vi "Process Messages.vi"(8 "error in (no error)":errorcluster, 11 "Deck in":refnum<class "Deck.lvclass">) -> (0 "error out":errorcluster, 3 "Deck out":refnum<class "Deck.lvclass">)   [LabVIEW 2018, in "Deck.lvclass"]
uses:
  Deck.lvclass
  Deck.lvclass/Deck.ctl
  State.ctl
  Libraries/Messaging/Message Cluster.ctl
  Libraries/Track Info/Track Info.ctl
  Libraries/Audio Processing/Value Properties.ctl
  Libraries/Track Info/Track Info FGV Enum.ctl
  d748f491-0a50-4902-99a1-0e4baec2160f.vi
  Libraries/Globals/Constants.vi
  Libraries/Audio Input/Audio File Input.lvlib
  Libraries/Messaging/Messaging.lvlib
  Libraries/User Interface/User Interface.lvlib
  Libraries/Track Info/Track Info.lvlib
  Libraries/Globals/Globals.lvlib
  Libraries/Audio Processing/Audio Processing.lvlib
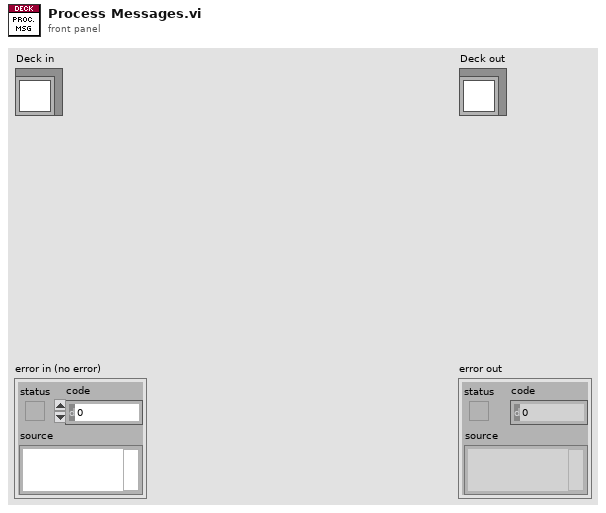
[diagram p1: front panel]
types:
  T1 = typedef "Messaging.lvlib/Message Cluster.ctl" = cluster{"Event":string, "Source":string, "Target":string, "Data":variant}
  T2 = typedef "Deck.lvclass/State.ctl" = enum16{"No Track", "Loading", "Active", "Scratching", "Brake", "Backspin"}
  T3 = typedef "Track Info.lvlib/Track Info.ctl" = cluster{"Path":path, "Length (Samples)":i32, "Channels":i32, "Sample Rate (Hz)":i32, "BPM":dbl, "Cue Points (Samples)":i32[]}
  T4 = typedef "Audio Processing.lvlib/Value Properties.ctl" = cluster{"Lower":dbl, "Upper":dbl}
  T5 = typedef "Track Info.lvlib/Track Info FGV Enum.ctl" = enum16{"Init", "Update Track", "Update Multiple Tracks", "Get Track", "Get Multiple Tracks"}
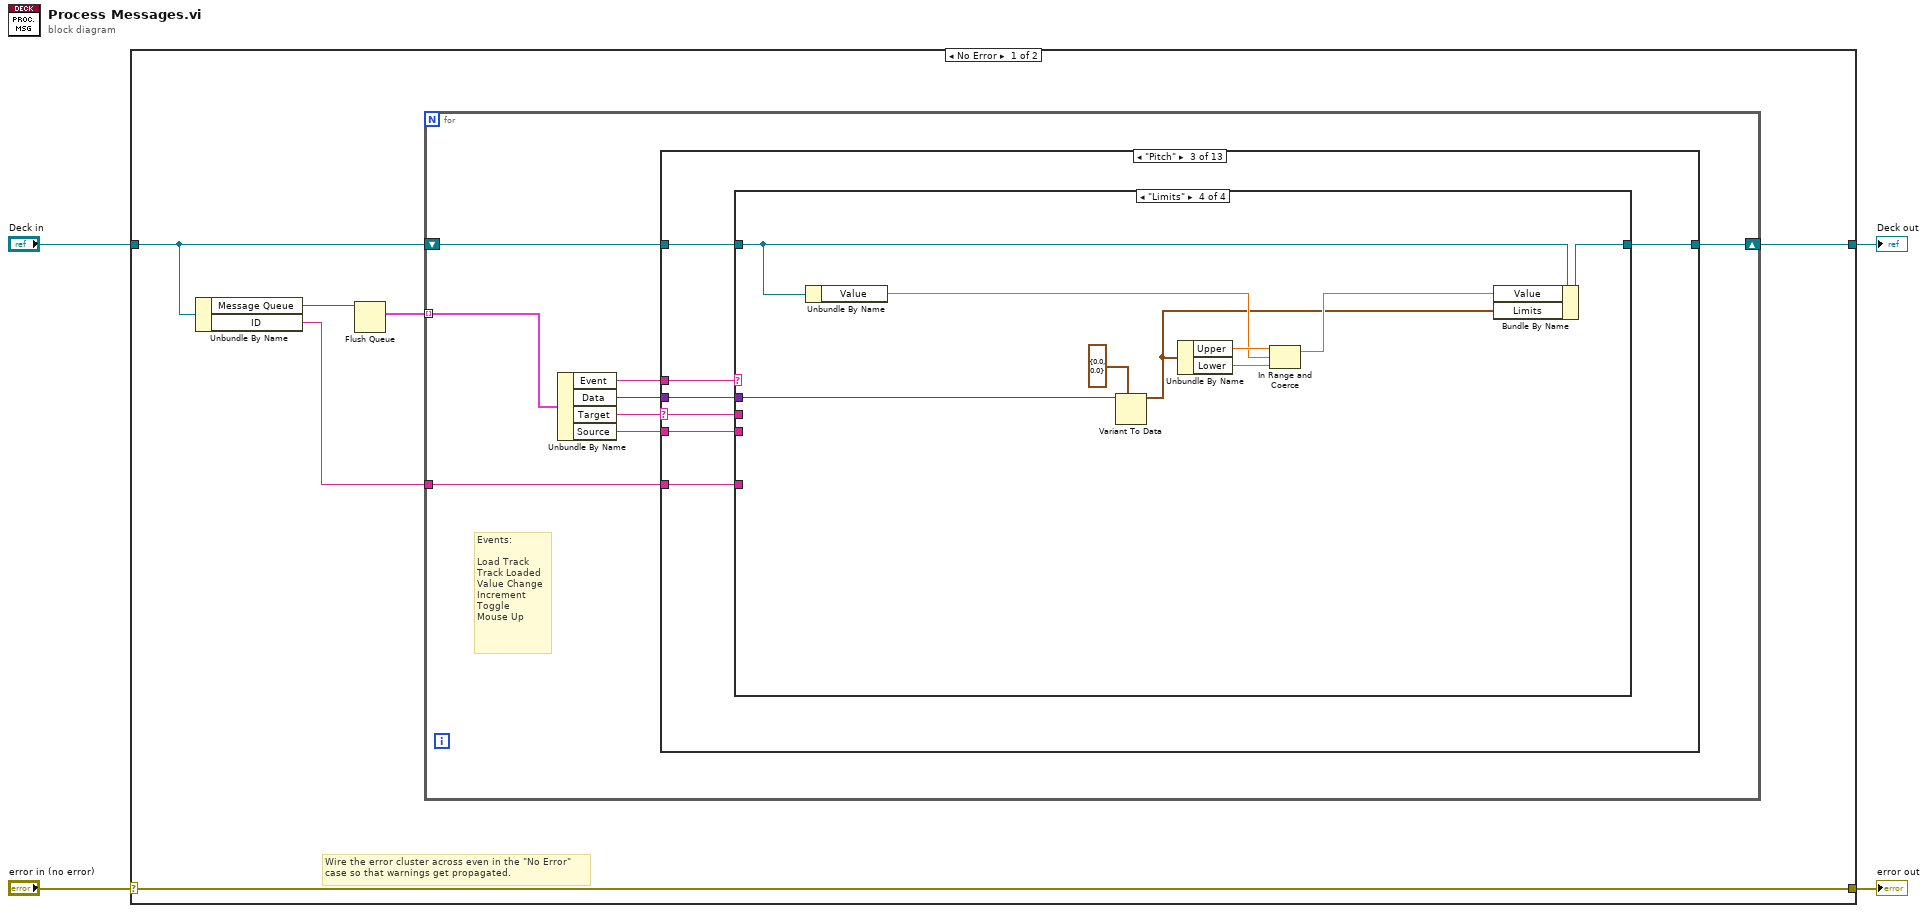
[diagram p0: block diagram]
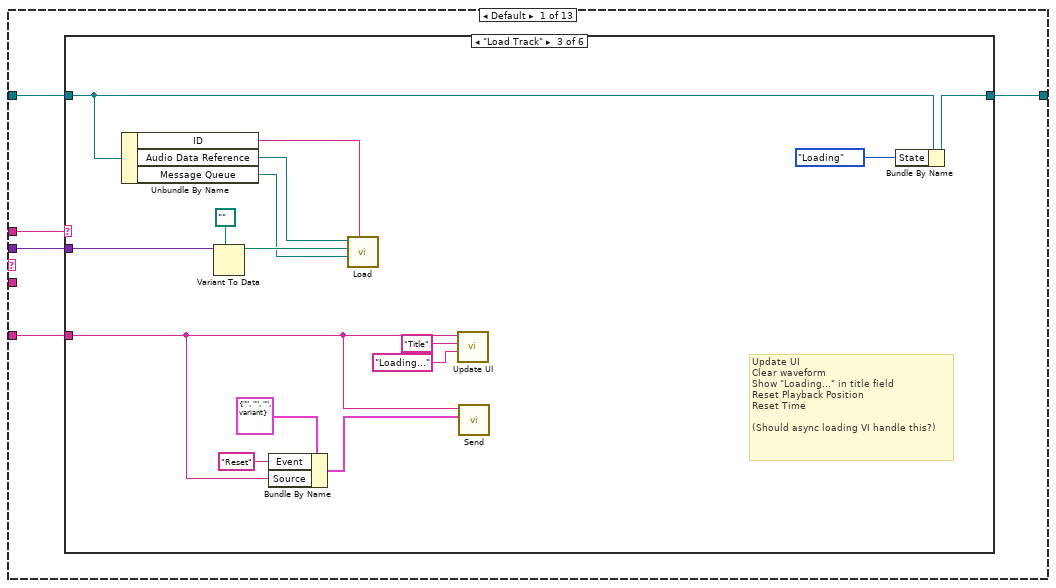
[diagram p2: hidden frame]
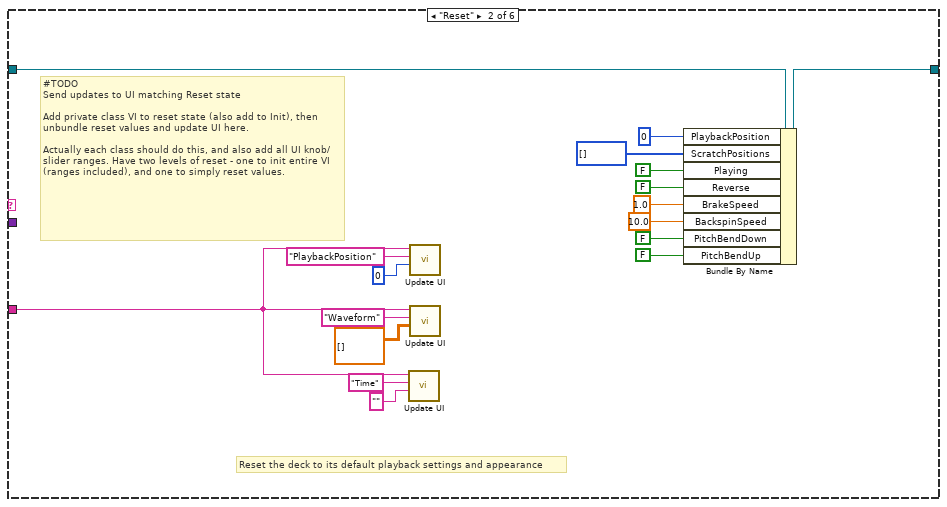
[diagram p4: hidden frame]
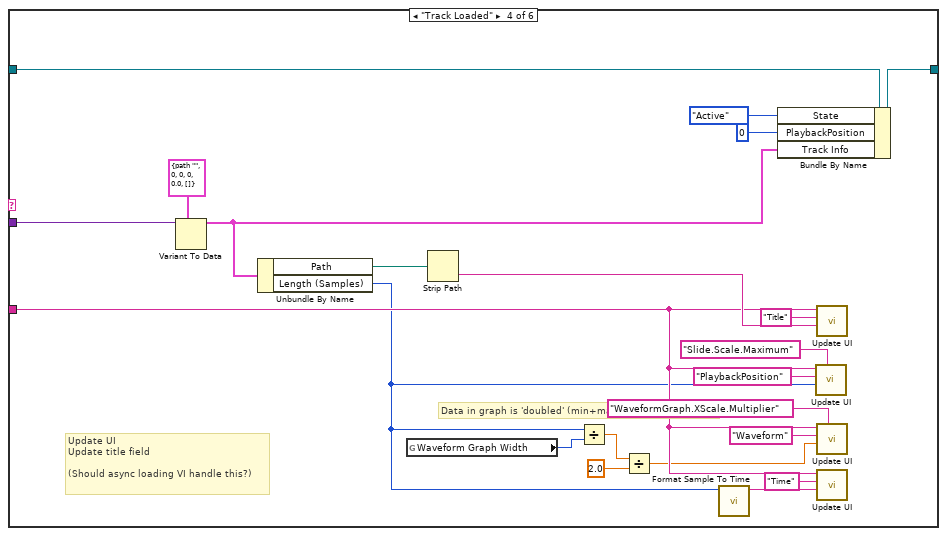
[diagram p5: hidden frame]
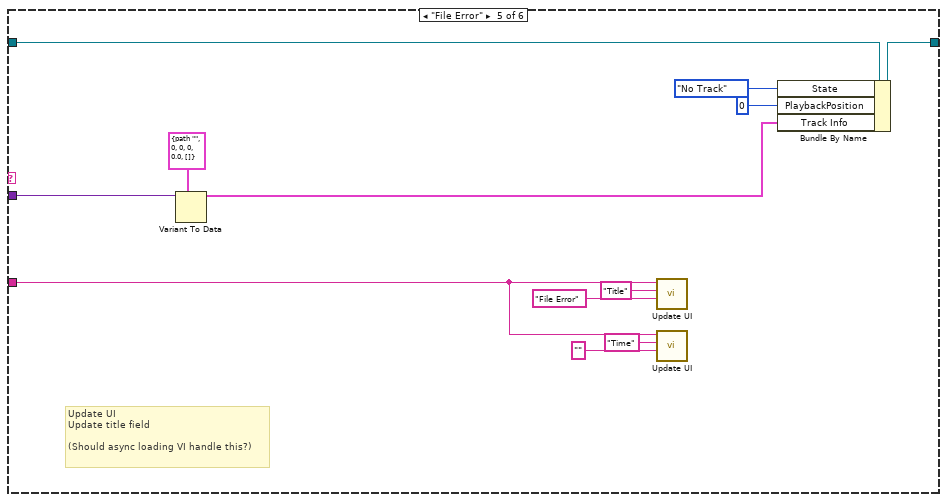
[diagram p6: hidden frame]
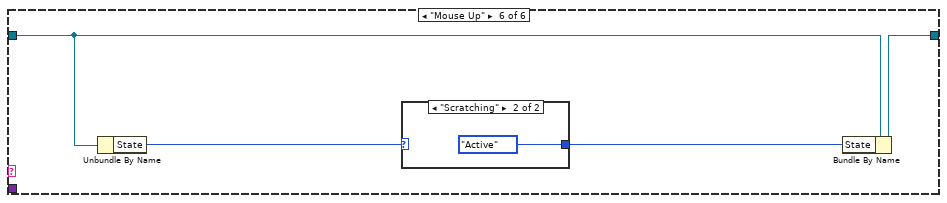
[diagram p7: hidden frame]
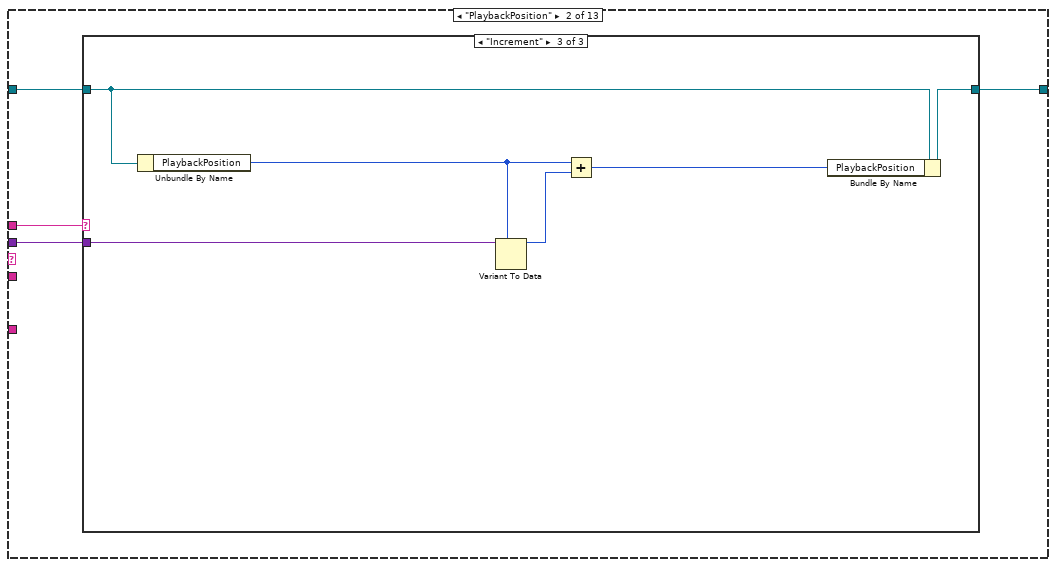
[diagram p9: hidden frame]
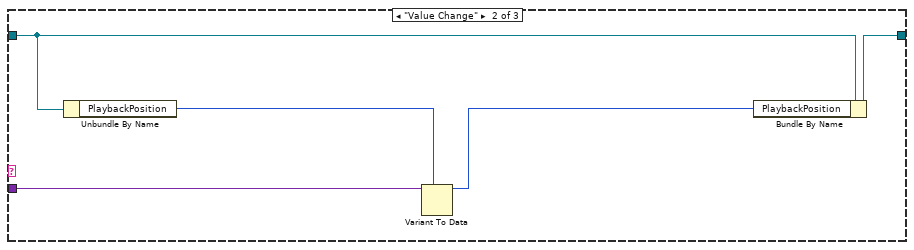
[diagram p11: hidden frame]
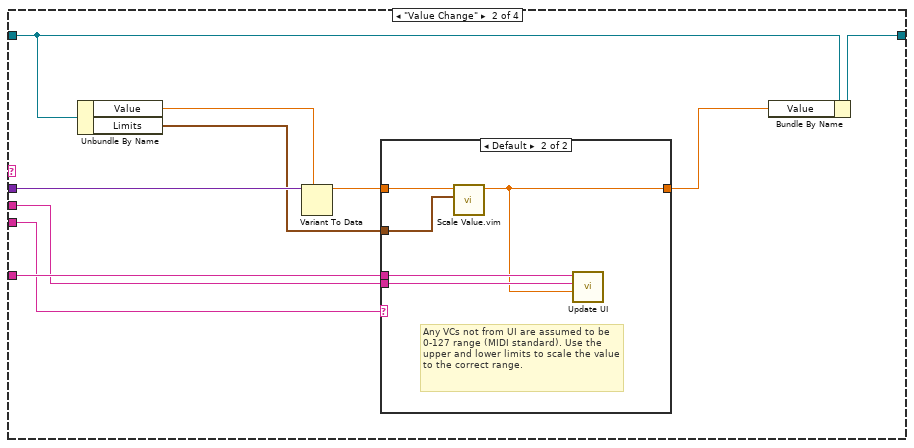
[diagram p13: hidden frame]
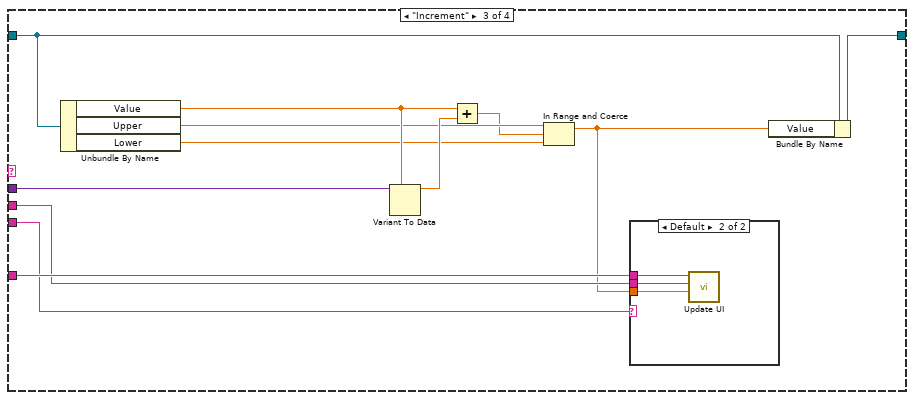
[diagram p15: hidden frame]
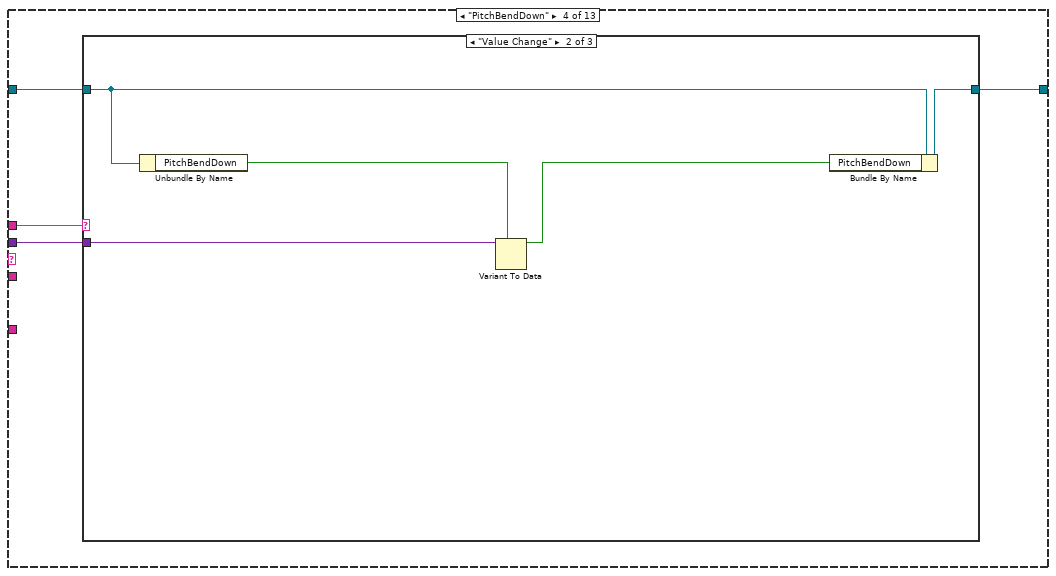
[diagram p17: hidden frame]
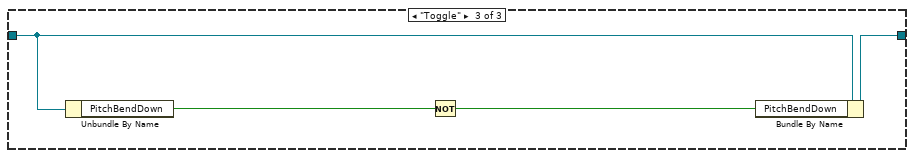
[diagram p19: hidden frame]
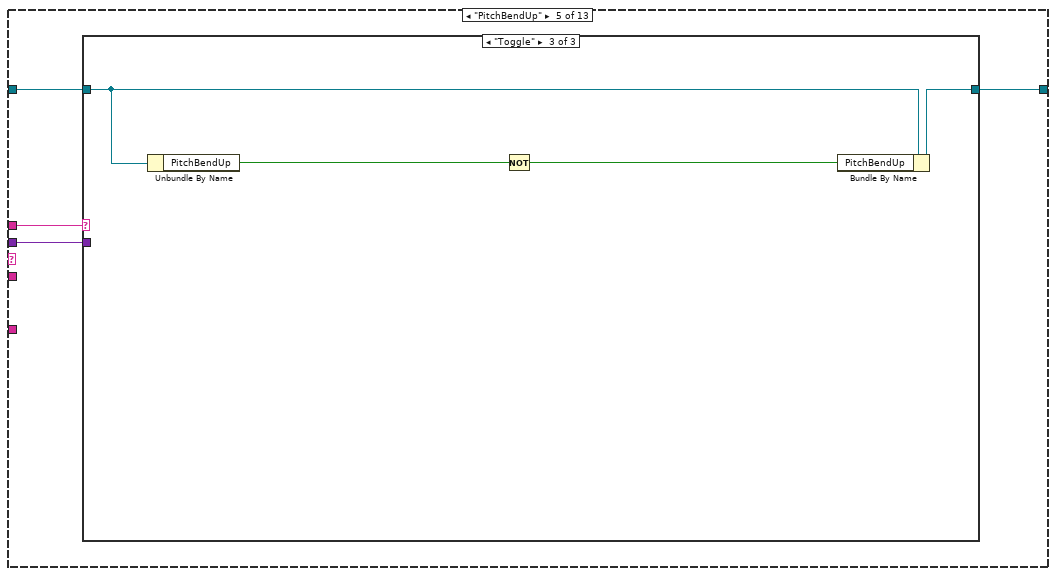
[diagram p20: hidden frame]
diagram:
  n1 = case shown="No Error" "error in (no error)" {
    selector: "error in (no error)" -> [w10 w528]
    tunnel: [w10 w528] -> w3
    tunnel: [w9 w527] -> w1
    tunnel: "Deck in" -> [w8 w527]
    frame No Error {
      # "Wire the error cluster across even in the \"No Error\"\ncase so that warnings get propagated."
      n2 = Unbundle By Name(w8) -> ("Message Queue"=w6:refnum<queue>, "ID"=w7:string)
      n3 = Flush Queue(queue=w6) -> (remaining elements=w5:T1[])  [unwired: 1 in, 2 out]
      n4 = for {
        shift-right: [w16] -> w9
        shift-left: w8 -> [w18]
        tunnel: w7 -> [w14]
        tunnel: w5 -> [w11] mode=indexing
        # "Events:\n\nLoad Track\nTrack Loaded\nValue Change\nIncrement\nToggle\nMouse Up"
        n5 = Unbundle By Name(w11) -> ("Event"=w17:string, "Data"=w15:variant, "Target"=w13:string, "Source"=w12:string)
        n6 = case shown="\"Pitch\"" w13 {
          selector: w13 -> [_ _ w114 _ _ _ w208 w239 w260 w280 w317 w347 w438]
          tunnel: w18 -> [w23 w100 w119 w164 w178 w192 w213 w243 w264 w284 w322 w351 w442]
          tunnel: w17 -> [w22 w99 w118 w163 w177 w191 w212 w242 w263 w283 w321 w350 w441]
          tunnel: [w21 w98 w117 w162 w176 w190 w211 w241 w262 w282 w320 w349 w440] -> w16
          tunnel: w15 -> [w20 w97 w116 w161 w175 w189 w210 w240 w261 w281 w319 w348 w439]
          tunnel: w14 -> [w19 _ w115 _ _ _ w209 w238 _ w279 w318 w346 w437]
          tunnel: w12 -> [_ _ w113 _ _ _ _ _ _ w278 w316 w345 w436]
          frame Default {
            n7 = case shown="\"Load Track\"" w22 {
              tunnel: w23 -> [w24 w33 w49 w76 w88 w91]
              tunnel: [w24 w34 w50 w75 w87 w92] -> w21
              tunnel: w20 -> [_ _ w48 w74 w86 _]
              tunnel: w19 -> [_ w35 w43 w62 w82 _]
              frame Default {
              }
              frame "Reset" {
                # "#TODO\nSend updates to UI matching Reset state\n\nAdd private class VI to reset state (also add to Init), then unbundle reset values and update UI here.\n\nActually each class should do this, and also add all UI knob/slider ranges. Have two levels of reset - one to init entire VI (ranges included), and one to simply reset values."
                # "Reset the deck to its default playback settings and appearance"
                n8 = call "Update UI.vi"("Data"="" ("Target"), "Target"="Time", "ID"=w35) -> ()  [unwired: 8 in, 1 out]
                n9 = call "Update UI.vi"("Data"=0, "Target"="PlaybackPosition", "ID"=w35) -> ()  [unwired: 8 in, 1 out]
                n10 = call "Update UI.vi"("Data"=dbl[][] [], "Target"="Waveform", "ID"=w35) -> ()  [unwired: 8 in, 1 out]
                n11 = Bundle By Name(cluster=w33, "PlaybackPosition"=0, "ScratchPositions"=i32[] [], "Playing"=FALSE, "Reverse"=FALSE, "BrakeSpeed"=1.0, "BackspinSpeed"=10.0, "PitchBendDown"=FALSE, "PitchBendUp"=FALSE) -> (w34:refnum<class "Deck.lvclass">)
              }
              frame "Load Track" {
                # "Update UI\nClear waveform\nShow \"Loading...\" in title field\nReset Playback Position\nReset Time\n\n(Should async loading VI handle this?)"
                n12 = Unbundle By Name(w49) -> ("ID"=w56:string, "Audio Data Reference"=w53:refnum<data-value>, "Message Queue"=w52:refnum<queue>)
                n13 = Variant To Data(type=path "", Variant=w48) -> (data=w55:path)  [unwired: 1 in, 1 out]
                n14 = Bundle By Name(cluster=T1 {"Event"="", "Source"="", "Target"="", "Data"=variant} ("Message"), "Event"="Reset", "Source"=w43) -> (w42:T1)
                n15 = call "Load.vi"("Deck ID"=w56, "Message Queue"=w52, "Path"=w55, "Audio Data Reference"=w53) -> ()  [unwired: 7 in, 1 out]
                n16 = call "Update UI.vi"("Data"="Loading..." ("Target"), "Target"="Title", "ID"=w43) -> ()  [unwired: 8 in, 1 out]
                n17 = call "Send.vi"("Message"=w42, "Queue Name"=w43) -> ()  [unwired: 9 in, 1 out]
                n18 = Bundle By Name(cluster=w49, "State"=State."Loading") -> (w50:refnum<class "Deck.lvclass">)
              }
              frame "Track Loaded" {
                # "Data in graph is 'doubled' (min+max for every point)"
                # "Update UI\nUpdate title field\n\n(Should async loading VI handle this?)"
                n19 = Variant To Data(type=T3 {"Path"=path "", "Length (Samples)"=0, "Channels"=0, "Sample Rate (Hz)"=0, "BPM"=0.0, "Cue Points (Samples)"=[]} ("Track Info"), Variant=w74) -> (data=w72:T3)  [unwired: 1 in, 1 out]
                n20 = Unbundle By Name(w72) -> ("Path"=w71:path, "Length (Samples)"=w61:i32)
                n21 = global read "Constants.vi" "Waveform Graph Width"() -> (w60:i32)
                n22 = Strip Path(path=w71) -> (name=w70:string)  [unwired: 1 out]
                n23 = Divide(x=w61, y=w60) -> (x/y=w59:dbl)
                n24 = Divide(x=w59, y=2.0 ("x")) -> (x/y=w57:dbl)
                n25 = call "Format Sample To Time.vi"("Samples"=w61) -> ("Formatted Time"=w66:string)  [unwired: 10 in]
                n26 = Bundle By Name(cluster=w76, "State"=State."Active", "PlaybackPosition"=0 ("Playback Position (Samples)"), "Track Info"=w72) -> (w75:refnum<class "Deck.lvclass">)
                n27 = call "Update UI.vi"("Message (Value Change)"="Slide.Scale.Maximum" ("Target"), "Data"=w61, "Target"="PlaybackPosition", "ID"=w62) -> ()  [unwired: 7 in, 1 out]
                n28 = call "Update UI.vi"("Data"=w70, "Target"="Title", "ID"=w62) -> ()  [unwired: 8 in, 1 out]
                n29 = call "Update UI.vi"("Message (Value Change)"="WaveformGraph.XScale.Multiplier" ("Target"), "Data"=w57, "Target"="Waveform", "ID"=w62) -> ()  [unwired: 7 in, 1 out]
                n30 = call "Update UI.vi"("Data"=w66, "Target"="Time", "ID"=w62) -> ()  [unwired: 8 in, 1 out]
              }
              frame "File Error" {
                # "Update UI\nUpdate title field\n\n(Should async loading VI handle this?)"
                n31 = Variant To Data(type=T3 {"Path"=path "", "Length (Samples)"=0, "Channels"=0, "Sample Rate (Hz)"=0, "BPM"=0.0, "Cue Points (Samples)"=[]} ("Track Info"), Variant=w86) -> (data=w84:T3)  [unwired: 1 in, 1 out]
                n32 = call "Update UI.vi"("Data"="File Error" ("Target"), "Target"="Title", "ID"=w82) -> ()  [unwired: 8 in, 1 out]
                n33 = call "Update UI.vi"("Data"="" ("Target"), "Target"="Time", "ID"=w82) -> ()  [unwired: 8 in, 1 out]
                n34 = Bundle By Name(cluster=w88, "State"=State."No Track", "PlaybackPosition"=0 ("Playback Position (Samples)"), "Track Info"=w84) -> (w87:refnum<class "Deck.lvclass">)
              }
              frame "Mouse Up" {
                n35 = Unbundle By Name(w91) -> ("State"=w93:T2)
                n36 = case shown="\"Scratching\"" w93 {
                  selector: w93 -> [w95 _]
                  tunnel: [w95 State."Active" ("State")] -> w94
                  frame Default {
                  }
                  frame "Scratching" {
                  }
                }
                n37 = Bundle By Name(cluster=w91, "State"=w94) -> (w92:refnum<class "Deck.lvclass">)
              }
            }
          }
          frame "PlaybackPosition" {
            n38 = case shown="\"Increment\"" w99 {
              tunnel: w100 -> [w101 w105 w111]
              tunnel: [w101 w106 w112] -> w98
              tunnel: w97 -> [_ w103 w110]
              frame Default {
              }
              frame "Value Change" {
                n39 = Unbundle By Name(w105) -> ("PlaybackPosition"=w104:i32)
                n40 = Variant To Data(type=w104, Variant=w103) -> (data=w102:i32)  [unwired: 1 in, 1 out]
                n41 = Bundle By Name(cluster=w105, "PlaybackPosition"=w102) -> (w106:refnum<class "Deck.lvclass">)
              }
              frame "Increment" {
                n42 = Unbundle By Name(w111) -> ("PlaybackPosition"=w109:i32)
                n43 = Variant To Data(type=w109, Variant=w110) -> (data=w108:i32)  [unwired: 1 in, 1 out]
                n44 = Add(x=w109, y=w108) -> (x+y=w107:i32)
                n45 = Bundle By Name(cluster=w111, "PlaybackPosition"=w107) -> (w112:refnum<class "Deck.lvclass">)
              }
            }
          }
          frame "Pitch" {
            n46 = case shown="\"Limits\"" w118 {
              tunnel: w119 -> [w120 w129 w147 w159]
              tunnel: [w120 w130 w148 w160] -> w117
              tunnel: w116 -> [_ w127 w146 w158]
              tunnel: w115 -> [_ w126 w143 _]
              tunnel: w114 -> [_ w124 w142 _]
              tunnel: w113 -> [_ w123 w141 _]
              frame Default {
              }
              frame "Value Change" {
                n47 = Unbundle By Name(w129) -> ("Value"=w128:dbl, "Limits"=w121:T4)
                n48 = Variant To Data(type=w128, Variant=w127) -> (data=w125:dbl)  [unwired: 1 in, 1 out]
                n49 = case shown="Default" w123 {
                  tunnel: w126 -> [_ w136]
                  tunnel: w124 -> [_ w135]
                  tunnel: w125 -> [w131 w132]
                  tunnel: [w131 w133] -> w122
                  tunnel: w121 -> [_ w134]
                  frame "UI" {
                    # "VC from UI are assumed to be in range."
                  }
                  frame Default {
                    # "Any VCs not from UI are assumed to be 0-127 range (MIDI standard). Use the upper and lower limits to scale the value to the correct range."
                    n50 = call "Scale Value.vim"("Limits"=w134, "Value"=w132) -> ("Scaled Value"=w133:dbl)  [unwired: 9 in]
                    n51 = call "Update UI.vi"("Data"=w133, "Target"=w135, "ID"=w136) -> ()  [unwired: 8 in, 1 out]
                  }
                }
                n52 = Bundle By Name(cluster=w129, "Value"=w122) -> (w130:refnum<class "Deck.lvclass">)
              }
              frame "Increment" {
                n53 = Unbundle By Name(w147) -> ("Value"=w145:dbl, "Upper"=w140:dbl, "Lower"=w139:dbl)
                n54 = Variant To Data(type=w145, Variant=w146) -> (data=w144:dbl)  [unwired: 1 in, 1 out]
                n55 = Add(x=w145, y=w144) -> (x+y=w138:dbl)
                n56 = In Range and Coerce(upper limit=w140, x=w138, lower limit=w139) -> (coerced(x)=w137:dbl)  [unwired: 1 out]
                n57 = case shown="Default" w141 {
                  tunnel: w143 -> [_ w151]
                  tunnel: w142 -> [_ w150]
                  tunnel: w137 -> [_ w149]
                  frame "UI" {
                  }
                  frame Default {
                    n58 = call "Update UI.vi"("Data"=w149, "Target"=w150, "ID"=w151) -> ()  [unwired: 8 in, 1 out]
                  }
                }
                n59 = Bundle By Name(cluster=w147, "Value"=w137) -> (w148:refnum<class "Deck.lvclass">)
              }
              frame "Limits" {
                n60 = Unbundle By Name(w159) -> ("Value"=w153:dbl)
                n61 = Variant To Data(type=T4 {"Lower"=0.0, "Upper"=0.0} ("Value Properties"), Variant=w158) -> (data=w152:T4)  [unwired: 1 in, 1 out]
                n62 = Unbundle By Name(w152) -> ("Upper"=w155:dbl, "Lower"=w154:dbl)
                n63 = In Range and Coerce(upper limit=w155, x=w153, lower limit=w154) -> (coerced(x)=w157:dbl)  [unwired: 1 out]
                n64 = Bundle By Name(cluster=w159, "Value"=w157, "Limits"=w152) -> (w160:refnum<class "Deck.lvclass">)
              }
            }
          }
          frame "PitchBendDown" {
            n65 = case shown="\"Value Change\"" w163 {
              tunnel: w164 -> [w165 w169 w173]
              tunnel: [w165 w170 w174] -> w162
              tunnel: w161 -> [_ w167 _]
              frame Default {
              }
              frame "Value Change" {
                n66 = Unbundle By Name(w169) -> ("PitchBendDown"=w168:bool)
                n67 = Variant To Data(type=w168, Variant=w167) -> (data=w166:bool)  [unwired: 1 in, 1 out]
                n68 = Bundle By Name(cluster=w169, "PitchBendDown"=w166) -> (w170:refnum<class "Deck.lvclass">)
              }
              frame "Toggle" {
                n69 = Unbundle By Name(w173) -> ("PitchBendDown"=w172:bool)
                n70 = Not(x=w172) -> (.not. x?=w171:bool)
                n71 = Bundle By Name(cluster=w173, "PitchBendDown"=w171) -> (w174:refnum<class "Deck.lvclass">)
              }
            }
          }
          frame "PitchBendUp" {
            n72 = case shown="\"Toggle\"" w177 {
              tunnel: w178 -> [w179 w183 w187]
              tunnel: [w179 w184 w188] -> w176
              tunnel: w175 -> [_ w181 _]
              frame Default {
              }
              frame "Value Change" {
                n73 = Unbundle By Name(w183) -> ("PitchBendUp"=w182:bool)
                n74 = Variant To Data(type=w182, Variant=w181) -> (data=w180:bool)  [unwired: 1 in, 1 out]
                n75 = Bundle By Name(cluster=w183, "PitchBendUp"=w180) -> (w184:refnum<class "Deck.lvclass">)
              }
              frame "Toggle" {
                n76 = Unbundle By Name(w187) -> ("PitchBendUp"=w186:bool)
                n77 = Not(x=w186) -> (.not. x?=w185:bool)
                n78 = Bundle By Name(cluster=w187, "PitchBendUp"=w185) -> (w188:refnum<class "Deck.lvclass">)
              }
            }
          }
          frame "Jogwheel" {
            n79 = case shown="\"Value Change\"" w191 {
              tunnel: w192 -> [w193 w204]
              tunnel: [w193 w205] -> w190
              tunnel: w189 -> [_ w203]
              frame Default {
              }
              frame "Value Change" {
                n80 = Unbundle By Name(w204) -> ("State"=w202:T2, "ScratchPositions"=w199:i32[], "PlaybackPosition"=w197:i32)
                n81 = Variant To Data(type=w197, Variant=w203) -> (data=w196:i32)  [unwired: 1 in, 1 out]
                n82 = Subtract(x=w199, y=w197) -> (x-y=w200:i32[])
                n83 = case shown="\"Active\"" w202 {
                  selector: w202 -> [w206 _]
                  tunnel: [w206 State."Scratching" ("State")] -> w201
                  frame Default {
                  }
                  frame "Active" {
                  }
                }
                n84 = Add Array Elements(numeric array=w200) -> (sum=w198:i32)
                n85 = Compound Arithmetic op=ADD(w198, w197, w196) -> (w195:i32)
                n86 = Build Array(w195) -> (w194:i32[])
                n87 = Bundle By Name(cluster=w204, "State"=w201, "ScratchPositions"=w194) -> (w205:refnum<class "Deck.lvclass">)
              }
            }
          }
          frame "Cue1", "Cue2", "Cue3" {
            n88 = case shown="\"Value Change\"" w212 {
              tunnel: w213 -> [w214 w225]
              tunnel: [w214 w226] -> w211
              tunnel: w210 -> [_ _]
              tunnel: w209 -> [_ w221]
              tunnel: w208 -> [_ w217]
              frame Default {
              }
              frame "Value Change" {
                n89 = Unbundle By Name(w225) -> ("Cue Points (Samples)"=w224:i32[], "Length (Samples)"=w220:i32)
                n90 = Reverse String(1:w217) -> (0:w219:string)
                n91 = Scan From String(format string="%d", input string=w219) -> (output 1=w216:i32)  [unwired: 3 in, 3 out]
                n92 = Decrement(x=w216) -> (x-1=w215:i32)
                n93 = Index Array(array=w224, index=w215) -> (element=w222:i32)
                n94 = Greater Or Equal To 0?(x=w222) -> (x >= 0?=w223:bool)
                n95 = case shown="True" w223 {
                  tunnel: [w227 w237] -> w226
                  tunnel: w225 -> [w227 w236]
                  tunnel: w222 -> [_ w229]
                  tunnel: w221 -> [_ w230]
                  tunnel: w220 -> [_ w231]
                  frame False {
                  }
                  frame True {
                    n96 = Subtract(x=w231, y=w229) -> (x-y=w228:i32)
                    n97 = call "Format Sample To Time.vi"("Samples"=w228) -> ("Formatted Time"=w235:string)  [unwired: 10 in]
                    n98 = Bundle By Name(cluster=w236, "PlaybackPosition"=w229) -> (w237:refnum<class "Deck.lvclass">)
                    n99 = call "Update UI.vi"("Data"=w229, "Target"="PlaybackPosition" ("format string"), "ID"=w230) -> ()  [unwired: 8 in, 1 out]
                    n100 = call "Update UI.vi"("Data"=w229, "Target"="Jogwheel" ("format string"), "ID"=w230) -> ()  [unwired: 8 in, 1 out]
                    n101 = call "Update UI.vi"("Data"=w235, "Target"="Time" ("format string"), "ID"=w230) -> ()  [unwired: 8 in, 1 out]
                  }
                }
              }
            }
          }
          frame "SetCue1", "SetCue2", "SetCue3" {
            n102 = case shown="\"Value Change\"" w242 {
              tunnel: w243 -> [w244 w259]
              tunnel: [w244 w255] -> w241
              tunnel: w240 -> [_ _]
              tunnel: w239 -> [_ w253]
              tunnel: w238 -> [_ w246]
              frame Default {
              }
              frame "Value Change" {
                n103 = Unbundle By Name(w259) -> ("PlaybackPosition"=w258:i32, "Cue Points (Samples)"=w254:i32[])
                n104 = Reverse String(1:w253) -> (0:w252:string)
                n105 = Scan From String(format string="%d", input string=w252) -> (output 1=w250:i32)  [unwired: 3 in, 3 out]
                n106 = Decrement(x=w250) -> (x-1=w249:i32)
                n107 = Replace Array Subset(array=w254, new element=w258, index=w249) -> (w247:i32[])
                n108 = Bundle By Name(cluster=w259, "Cue Points (Samples)"=w247) -> (w255:refnum<class "Deck.lvclass">)
                n109 = call "Update UI.vi"("Message (Value Change)"="WaveformGraph.Cues" ("format string"), "Data"=w247, "Target"="Waveform", "ID"=w246) -> ()  [unwired: 7 in, 1 out]
                n110 = Unbundle By Name(w255) -> ("Track Info"=w257:T3)
                n111 = call "Track Info FGV.vi"("Track Info FGV Enum"=Track_Info_FGV_Enum."Update Track", "Track Info In"=w257) -> ()  [unwired: 6 in, 4 out]
              }
            }
          }
          frame "ClearCue1", "ClearCue2", "ClearCue3" {
            n112 = case shown="\"Value Change\"" w263 {
              tunnel: w264 -> [w265 w277]
              tunnel: [w265 w266] -> w262
              tunnel: w261 -> [_ _]
              tunnel: w260 -> [_ w269]
              frame Default {
              }
              frame "Value Change" {
                n113 = Unbundle By Name(w277) -> ("Cue Points (Samples)"=w276:i32[])
                n114 = Reverse String(1:w269) -> (0:w271:string)
                n115 = Scan From String(format string="%d", input string=w271) -> (output 1=w268:i32)  [unwired: 3 in, 3 out]
                n116 = Decrement(x=w268) -> (x-1=w267:i32)
                n117 = Replace Array Subset(array=w276, new element=-2147483648 ("new element/subarray"), index=w267) -> (w275:i32[])
                n118 = Bundle By Name(cluster=w277, "Cue Points (Samples)"=w275) -> (w266:refnum<class "Deck.lvclass">)
                n119 = Unbundle By Name(w266) -> ("Track Info"=w273:T3)
                n120 = call "Track Info FGV.vi"("Track Info FGV Enum"=Track_Info_FGV_Enum."Update Track", "Track Info In"=w273) -> ()  [unwired: 6 in, 4 out]
              }
            }
          }
          frame "Play" {
            n121 = case shown="\"Value Change\"" w283 {
              tunnel: w284 -> [w285 w293 w308]
              tunnel: [w285 w294 w309] -> w282
              tunnel: w281 -> [_ w291 _]
              tunnel: w280 -> [_ w289 w305]
              tunnel: w279 -> [_ w288 w304]
              tunnel: w278 -> [_ w287 w302]
              frame Default {
              }
              frame "Value Change" {
                n122 = Unbundle By Name(w293) -> ("State"=w292:T2, "Playing"=w290:bool)
                n123 = case shown="Default" w292 {
                  tunnel: w291 -> [_ w301]
                  tunnel: w290 -> [w298 w300]
                  tunnel: [w298 w299] -> w286
                  frame Default {
                  }
                  frame "Active".."Backspin" {
                    n124 = Variant To Data(type=w300, Variant=w301) -> (data=w299:bool)  [unwired: 1 in, 1 out]
                  }
                }
                n125 = case shown="Default" w287 {
                  tunnel: w288 -> [_ w297]
                  tunnel: w289 -> [_ w296]
                  tunnel: w286 -> [_ w295]
                  frame "UI" {
                  }
                  frame Default {
                    n126 = call "Update UI.vi"("Data"=w295, "Target"=w296, "ID"=w297) -> ()  [unwired: 8 in, 1 out]
                  }
                }
                n127 = Bundle By Name(cluster=w293, "Playing"=w286) -> (w294:refnum<class "Deck.lvclass">)
              }
              frame "Toggle" {
                n128 = Unbundle By Name(w308) -> ("State"=w307:T2, "Playing"=w306:bool)
                n129 = case shown="Default" w307 {
                  tunnel: w306 -> [w313 w315]
                  tunnel: [w313 w314] -> w303
                  frame Default {
                  }
                  frame "Active".."Backspin" {
                    n130 = Not(x=w315) -> (.not. x?=w314:bool)
                  }
                }
                n131 = case shown="Default" w302 {
                  tunnel: w304 -> [_ w312]
                  tunnel: w305 -> [_ w311]
                  tunnel: w303 -> [_ w310]
                  frame "UI" {
                  }
                  frame Default {
                    n132 = call "Update UI.vi"("Data"=w310, "Target"=w311, "ID"=w312) -> ()  [unwired: 8 in, 1 out]
                  }
                }
                n133 = Bundle By Name(cluster=w308, "Playing"=w303) -> (w309:refnum<class "Deck.lvclass">)
              }
            }
          }
          frame "Reverse" {
            n134 = case shown="\"Value Change\"" w321 {
              tunnel: w322 -> [w323 w330 w340]
              tunnel: [w323 w331 w341] -> w320
              tunnel: w319 -> [_ w329 _]
              tunnel: w318 -> [_ w327 w337]
              tunnel: w317 -> [_ w326 w336]
              tunnel: w316 -> [_ w325 w335]
              frame Default {
              }
              frame "Value Change" {
                n135 = Unbundle By Name(w330) -> ("Reverse"=w328:bool)
                n136 = Variant To Data(type=w328, Variant=w329) -> (data=w324:bool)  [unwired: 1 in, 1 out]
                n137 = case shown="Default" w325 {
                  tunnel: w327 -> [_ w334]
                  tunnel: w326 -> [_ w333]
                  tunnel: w324 -> [_ w332]
                  frame "UI" {
                  }
                  frame Default {
                    n138 = call "Update UI.vi"("Data"=w332, "Target"=w333, "ID"=w334) -> ()  [unwired: 8 in, 1 out]
                  }
                }
                n139 = Bundle By Name(cluster=w330, "Reverse"=w324) -> (w331:refnum<class "Deck.lvclass">)
              }
              frame "Toggle" {
                n140 = Unbundle By Name(w340) -> ("Reverse"=w339:bool)
                n141 = Not(x=w339) -> (.not. x?=w338:bool)
                n142 = case shown="Default" w335 {
                  tunnel: w337 -> [_ w344]
                  tunnel: w336 -> [_ w343]
                  tunnel: w338 -> [_ w342]
                  frame "UI" {
                  }
                  frame Default {
                    n143 = call "Update UI.vi"("Data"=w342, "Target"=w343, "ID"=w344) -> ()  [unwired: 8 in, 1 out]
                  }
                }
                n144 = Bundle By Name(cluster=w340, "Reverse"=w338) -> (w341:refnum<class "Deck.lvclass">)
              }
            }
          }
          frame "Brake" {
            n145 = case shown="\"Toggle\"" w350 {
              tunnel: w351 -> [w352 w365 w414]
              tunnel: [w352 w366 w415] -> w349
              tunnel: w348 -> [_ w361 _]
              tunnel: w347 -> [_ w357 w409]
              tunnel: w346 -> [_ w356 w408]
              tunnel: w345 -> [_ _ _]
              frame Default {
              }
              frame "Value Change" {
                n146 = Unbundle By Name(w365) -> ("Playing"=w358:bool, "State"=w359:T2, "BrakeSpeed"=w364:dbl)
                n147 = Variant To Data(type=FALSE, Variant=w361) -> (data=w360:bool)  [unwired: 1 in, 1 out]
                n148 = case shown="\"Brake\"" w359 {
                  selector: w359 -> [w367 w369 w387]
                  tunnel: w360 -> [_ w371 w389]
                  tunnel: w364 -> [w368 w372 w390]
                  tunnel: [w368 w373 w391] -> w363
                  tunnel: [w367 w374 w392] -> w355
                  tunnel: w358 -> [_ w370 w388]
                  frame Default {
                  }
                  frame "Active" {
                    n149 = case shown="True" w370 {
                      selector: w370 -> [_ w379]
                      tunnel: [w375 w382] -> w374
                      tunnel: [w376 w381] -> w373
                      tunnel: w372 -> [w376 w380]
                      tunnel: w371 -> [_ w378]
                      tunnel: w369 -> [w375 w377]
                      frame False {
                      }
                      frame True {
                        n150 = case shown="True" w378 {
                          tunnel: [w383 State."Brake" ("State")] -> w382
                          tunnel: [w384 1.0 ("BrakeSpeed")] -> w381
                          tunnel: w380 -> [w384 _]
                          tunnel: w379 -> [_ _]
                          tunnel: w377 -> [w383 _]
                          frame False {
                          }
                          frame True {
                          }
                        }
                      }
                    }
                  }
                  frame "Brake" {
                    n151 = case shown="True" w388 {
                      selector: w388 -> [_ w397]
                      tunnel: [w393 w400] -> w392
                      tunnel: [w394 w399] -> w391
                      tunnel: w390 -> [w394 w398]
                      tunnel: w389 -> [_ w396]
                      tunnel: w387 -> [w393 w395]
                      frame False {
                      }
                      frame True {
                        n152 = case shown="False" w396 {
                          tunnel: [State."Active" ("State") w403] -> w400
                          tunnel: [1.0 ("BrakeSpeed") w404] -> w399
                          tunnel: w398 -> [_ w404]
                          tunnel: w397 -> [_ _]
                          tunnel: w395 -> [_ w403]
                          frame False {
                          }
                          frame True {
                          }
                        }
                      }
                    }
                  }
                }
                n153 = Equal?(x=w355, y=State."Brake") -> (x = y?=w353:bool)
                n154 = Bundle By Name(cluster=w365, "State"=w355, "BrakeSpeed"=w363) -> (w366:refnum<class "Deck.lvclass">)
                n155 = call "Update UI.vi"("Data"=w353, "Target"=w357, "ID"=w356) -> ()  [unwired: 8 in, 1 out]
              }
              frame "Toggle" {
                n156 = Unbundle By Name(w414) -> ("Playing"=w410:bool, "State"=w411:T2, "BrakeSpeed"=w413:dbl)
                n157 = case shown="\"Active\"" w411 {
                  selector: w411 -> [w416 w418 w427]
                  tunnel: w413 -> [w417 w420 w429]
                  tunnel: [w417 w421 w430] -> w412
                  tunnel: [w416 w422 w431] -> w407
                  tunnel: w410 -> [_ w419 w428]
                  frame Default {
                  }
                  frame "Active" {
                    n158 = case shown="True" w419 {
                      tunnel: [w423 State."Brake" ("State")] -> w422
                      tunnel: [w424 1.0 ("BrakeSpeed")] -> w421
                      tunnel: w420 -> [w424 _]
                      tunnel: w418 -> [w423 _]
                      frame False {
                      }
                      frame True {
                      }
                    }
                  }
                  frame "Brake" {
                    n159 = case shown="True" w428 {
                      tunnel: [w432 State."Active" ("State")] -> w431
                      tunnel: [w433 1.0 ("BrakeSpeed")] -> w430
                      tunnel: w429 -> [w433 _]
                      tunnel: w427 -> [w432 _]
                      frame False {
                      }
                      frame True {
                      }
                    }
                  }
                }
                n160 = Equal?(x=w407, y=State."Brake" ("State")) -> (x = y?=w405:bool)
                n161 = Bundle By Name(cluster=w414, "State"=w407, "BrakeSpeed"=w412) -> (w415:refnum<class "Deck.lvclass">)
                n162 = call "Update UI.vi"("Data"=w405, "Target"=w409, "ID"=w408) -> ()  [unwired: 8 in, 1 out]
              }
            }
          }
          frame "Backspin" {
            n163 = case shown="\"Toggle\"" w441 {
              tunnel: w442 -> [w443 w456 w505]
              tunnel: [w443 w457 w506] -> w440
              tunnel: w439 -> [_ w452 _]
              tunnel: w438 -> [_ w448 w500]
              tunnel: w437 -> [_ w447 w499]
              tunnel: w436 -> [_ _ _]
              frame Default {
              }
              frame "Value Change" {
                n164 = Unbundle By Name(w456) -> ("Playing"=w449:bool, "State"=w450:T2, "BackspinSpeed"=w455:dbl)
                n165 = Variant To Data(type=FALSE, Variant=w452) -> (data=w451:bool)  [unwired: 1 in, 1 out]
                n166 = case shown="\"Backspin\"" w450 {
                  selector: w450 -> [w458 w460 w478]
                  tunnel: w451 -> [_ w462 w480]
                  tunnel: w455 -> [w459 w463 w481]
                  tunnel: [w459 w464 w482] -> w454
                  tunnel: [w458 w465 w483] -> w446
                  tunnel: w449 -> [_ w461 w479]
                  frame Default {
                  }
                  frame "Active" {
                    n167 = case shown="True" w461 {
                      selector: w461 -> [_ w470]
                      tunnel: [w466 w473] -> w465
                      tunnel: [w467 w472] -> w464
                      tunnel: w463 -> [w467 w471]
                      tunnel: w462 -> [_ w469]
                      tunnel: w460 -> [w466 w468]
                      frame False {
                      }
                      frame True {
                        n168 = case shown="True" w469 {
                          tunnel: [w474 State."Backspin" ("State")] -> w473
                          tunnel: [w475 5.0 ("BrakeSpeed")] -> w472
                          tunnel: w471 -> [w475 _]
                          tunnel: w470 -> [_ _]
                          tunnel: w468 -> [w474 _]
                          frame False {
                          }
                          frame True {
                          }
                        }
                      }
                    }
                  }
                  frame "Backspin" {
                    n169 = case shown="True" w479 {
                      selector: w479 -> [_ w488]
                      tunnel: [w484 w491] -> w483
                      tunnel: [w485 w490] -> w482
                      tunnel: w481 -> [w485 w489]
                      tunnel: w480 -> [_ w487]
                      tunnel: w478 -> [w484 w486]
                      frame False {
                      }
                      frame True {
                        n170 = case shown="False" w487 {
                          tunnel: [State."Active" ("State") w494] -> w491
                          tunnel: [5.0 ("BrakeSpeed") w495] -> w490
                          tunnel: w489 -> [_ w495]
                          tunnel: w488 -> [_ _]
                          tunnel: w486 -> [_ w494]
                          frame False {
                          }
                          frame True {
                          }
                        }
                      }
                    }
                  }
                }
                n171 = Equal?(x=w446, y=State."Backspin") -> (x = y?=w444:bool)
                n172 = Bundle By Name(cluster=w456, "State"=w446, "BackspinSpeed"=w454) -> (w457:refnum<class "Deck.lvclass">)
                n173 = call "Update UI.vi"("Data"=w444, "Target"=w448, "ID"=w447) -> ()  [unwired: 8 in, 1 out]
              }
              frame "Toggle" {
                n174 = Unbundle By Name(w505) -> ("Playing"=w501:bool, "State"=w502:T2, "BackspinSpeed"=w504:dbl)
                n175 = case shown="\"Active\"" w502 {
                  selector: w502 -> [w507 w509 w518]
                  tunnel: w504 -> [w508 w511 w520]
                  tunnel: [w508 w512 w521] -> w503
                  tunnel: [w507 w513 w522] -> w498
                  tunnel: w501 -> [_ w510 w519]
                  frame Default {
                  }
                  frame "Active" {
                    n176 = case shown="True" w510 {
                      tunnel: [w514 State."Backspin" ("State")] -> w513
                      tunnel: [w515 5.0 ("BrakeSpeed")] -> w512
                      tunnel: w511 -> [w515 _]
                      tunnel: w509 -> [w514 _]
                      frame False {
                      }
                      frame True {
                      }
                    }
                  }
                  frame "Backspin" {
                    n177 = case shown="True" w519 {
                      tunnel: [w523 State."Active" ("State")] -> w522
                      tunnel: [w524 5.0 ("BrakeSpeed")] -> w521
                      tunnel: w520 -> [w524 _]
                      tunnel: w518 -> [w523 _]
                      frame False {
                      }
                      frame True {
                      }
                    }
                  }
                }
                n178 = Equal?(x=w498, y=State."Backspin" ("State")) -> (x = y?=w496:bool)
                n179 = Bundle By Name(cluster=w505, "State"=w498, "BackspinSpeed"=w503) -> (w506:refnum<class "Deck.lvclass">)
                n180 = call "Update UI.vi"("Data"=w496, "Target"=w500, "ID"=w499) -> ()  [unwired: 8 in, 1 out]
              }
            }
          }
        }
      }
    }
    frame Error {
    }
  }
  "error out" <- w3
  "Deck out" <- w1
